vi "gemv - General Matrix-Vector Product.vi"   [LabVIEW 2020, in "NI_AALBLAS.lvlib"]
doc: "Calculates the product of a general matrix and a vector."
uses:
  NI_AALBLAS.lvlib
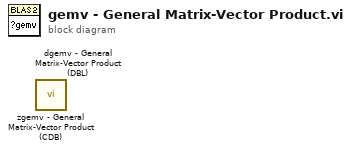
[diagram p0: block diagram]
diagram:
  n1 = call "zgemv - General Matrix-Vector Product (CDB).vi"() -> ()  [unwired: 10 in, 2 out]
  n2 = call "dgemv - General Matrix-Vector Product (DBL).vi"() -> ()  [unwired: 10 in, 2 out]
